vi "Autonomous Independent.vi"() -> ()   [LabVIEW 2020]
doc: "This VI is called when autonomous begins, and will automatically be terminated when autonomous ends. You can carry out timed or sensor driven robot movement independently without needing to return to the caller."
uses:
  <vilib>/Rock Robotics/WPI/Utilities/WPI_GetSetVariantRefNum.vi
  <vilib>/Rock Robotics/Network Tables/NT Write Numeric Array.vi
  Robot Global Data.vi
  <vilib>/Rock Robotics/Network Tables/NT Read String.vi
  <vilib>/Rock Robotics/WPI/RobotDrive/WPI_RobotDriveArcadeDrive_Standard(NoSaturation).vi
  <vilib>/Rock Robotics/WPI/ThirdParty/JAS_Junk/TrajLib/Trajectory_Library.lvlib
panel:
  out "Current Movement, for debugging":T1 {"Y Joystick Value" scale=1.0..-1.0; "X Joystick Value" scale=-1.0..1.0}
  in  "Array of robot movements":T2(array[cluster])=[{"X Joystick Value"=0.39393939393939403, "Y Joystick Value"=0.0, "Delay (sec)"=1.0, "Movement Name"="turn"}, {"X Joystick Value"=-0.3737373737373737, "Y Joystick Value"=0.0, "Delay (sec)"=1.0, "Movement Name"="turn back"}] {"Y Joystick Value" scale=1.0..-1.0; "X Joystick Value" scale=-1.0..1.0}
  # "Be sure to right-click and choose Data Operations>>Make Current Value default if you want to save the array values with the VI"
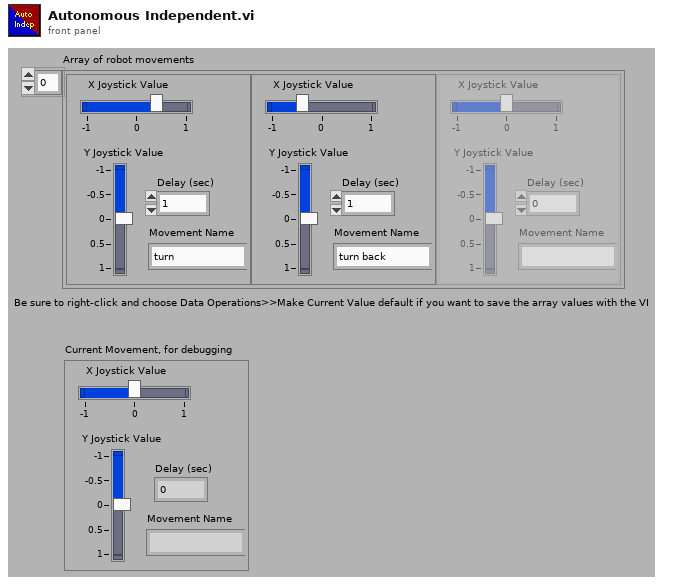
[diagram p1: front panel]
types:
  T1 = cluster{"X Joystick Value":dbl, "Y Joystick Value":dbl, "Delay (sec)":dbl, "Movement Name":string}
  T2 = cluster{"X Joystick Value":dbl, "Y Joystick Value":dbl, "Delay (sec)":dbl, "Movement Name":string}[]
  T3 = typedef "WPI_JoystickDevRef.ctl" = cluster{"Device":T4}
  T4 = typedef "WPI_JoystickDeviceEnum.ctl" = enum16{"USB 0", "USB 1", "USB 2", "USB 3", "USB 4", "USB 5"}
  T5 = typedef "Trajectory_Library.lvlib/SWERVE_DRIVE_ODOMETRY.ctl" = cluster{"POSE":T6, "GyroOffset":T8, "PreviousAngle":T8, "PrevModulePositions":T9[], "NumModules":i32}
  T6 = typedef "Trajectory_Library.lvlib/POSE2D.ctl" = cluster{"TRANSLATION":T7, "ROTATION":T8}
  T7 = typedef "Trajectory_Library.lvlib/TRANSLATION2D.ctl" = cluster{"X":dbl, "Y":dbl}
  T8 = typedef "Trajectory_Library.lvlib/ROTATION2D.ctl" = cluster{"VALUE":dbl, "COS":dbl, "SIN":dbl}
  T9 = typedef "Trajectory_Library.lvlib/SWERVE_DRIVE_MODULE_POSITION.ctl" = cluster{"Distance":dbl, "Angle":T8, "P":bool}
  T10 = typedef "WPI_RobotDriveDevRef.ctl" = cluster{"DevStatus":errorcluster, "Motors[]":T11[], "Square Inputs":bool, "Max Output":dbl}
  T11 = typedef "WPI_MotorControlDeviceRef.ctl" = cluster{"DeviceStatus":errorcluster, "Type":T12, "PWM":cluster{"PWM Channel":T13, "DeadBand":T14}, "CAN":cluster{"Device Number":u8, "SetOutput VI Ref":variant, "GetOutput VI Ref":variant, "Enable VI Ref":variant, "Disable VI Ref":variant, "Data":variant}, "Invert":bool, "DIO PWM":cluster{"PWM \"Enable\" Channel":T13, "DIOChannel":T15, "PWM Rate":dbl}}
  T12 = typedef "WPI_MotorControlType.ctl" = enum16{"PWM", "CAN", "DIO PWM"}
  T13 = typedef "FPGA_DIOPWMChannel.ctl" = enum8{"PWM 0", "PWM 1", "PWM 2", "PWM 3", "PWM 4", "PWM 5", "PWM 6", "PWM 7", "PWM 8", "PWM 9", "PWM MXP 0", "PWM MXP 1", "PWM MXP 2", "PWM MXP 3", "PWM MXP 4", "PWM MXP 5", "PWM MXP 6", "PWM MXP 7", "PWM MXP 8", "PWM MXP 9", "Invalid"}
  T14 = typedef "WPI_PWMDeadband.ctl" = cluster{"Name":string, "maxPositivePwm":i32, "minPositivePwm":i32, "centerPwm":i32, "maxNegativePwm":i32, "minNegativePwm":i32, "angularRange":u16}
  T15 = typedef "FPGA_DIOChannel.ctl" = enum8{"DIO 0", "DIO 1", "DIO 2", "DIO 3", "DIO 4", "DIO 5", "DIO 6", "DIO 7", "DIO 8", "DIO 9", "DIO MXP 0", "DIO MXP 1", "DIO MXP 2", "DIO MXP 3", "DIO MXP 4", "DIO MXP 5", "DIO MXP 6", "DIO MXP 7", "DIO MXP 8", "DIO MXP 9", "DIO MXP 10", "DIO MXP 11", "DIO MXP 12", "DIO MXP 13", "DIO MXP 14", "DIO MXP 15", "SPI Port CS1", "SPI Port CS2", "SPI Port CS3", "SPI Port MISO", "SPI Port MOSI", "Invalid"}
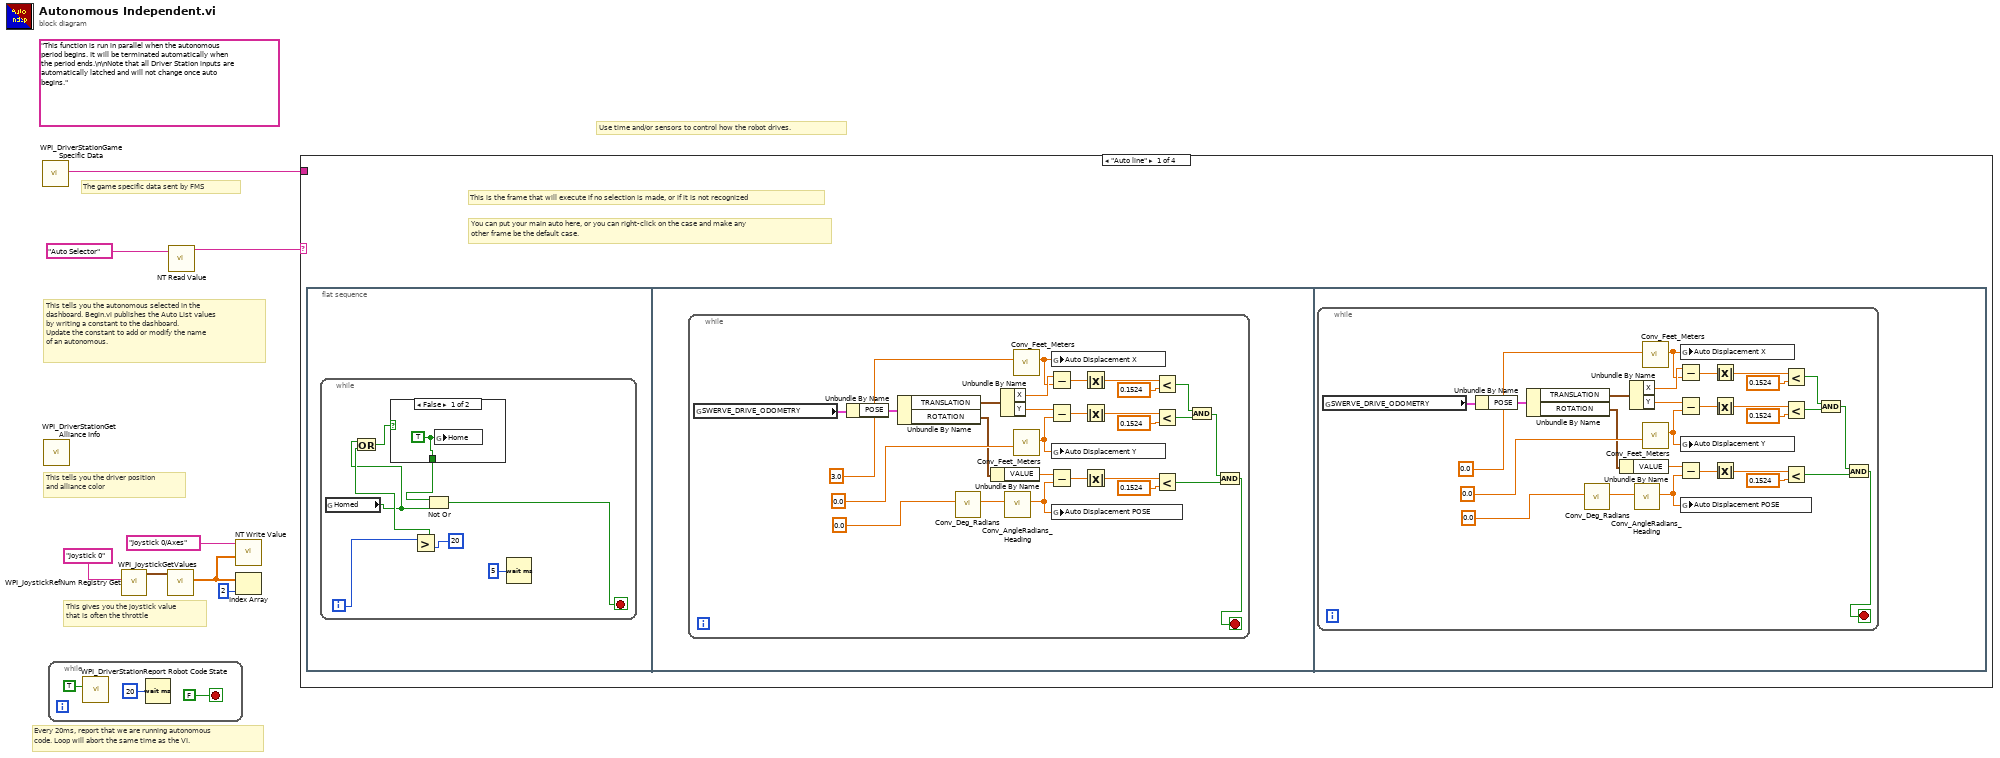
[diagram p0: block diagram]
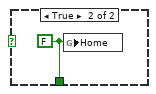
[diagram p2: hidden frame]
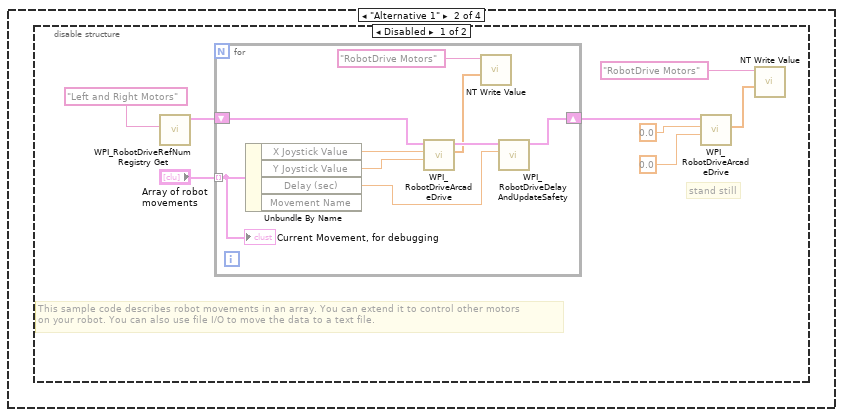
[diagram p3: hidden frame]
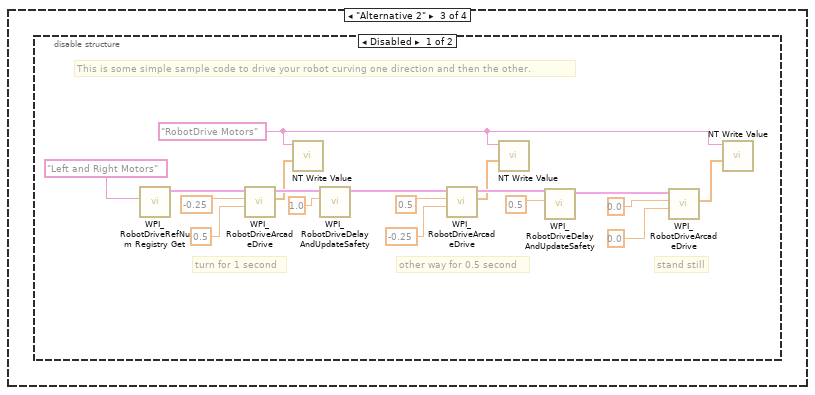
[diagram p5: hidden frame]
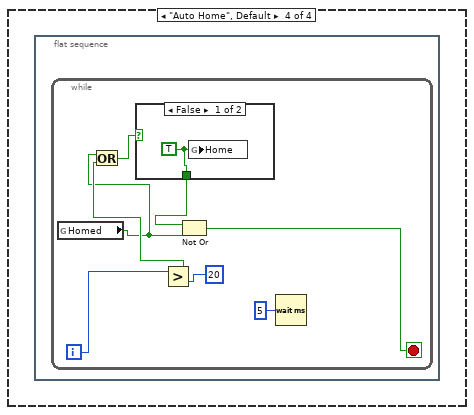
[diagram p7: hidden frame]
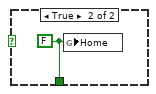
[diagram p8: hidden frame]
diagram:
  (unwired) "This function is run in parallel when the autonomous period begins. It will be terminated automatically when the period ends.\n\nNote that all Driver Station inputs are automatically latched and will not change once auto begins."
  # "The game specific data sent by FMS"
  # "This tells you the autonomous selected in the \ndashboard. Begin.vi publishes the Auto List values\nby writing a constant to the dashboard.\nUpdate the constant to add or modify the name\nof an autonomous."
  # "Every 20ms, report that we are running autonomous\ncode. Loop will abort the same time as the VI."
  # "This gives you the joystick value\nthat is often the throttle"
  # "Use time and/or sensors to control how the robot drives."
  # "This tells you the driver position\nand alliance color"
  n1 = call <vilib>:"WPI_DriverStationGame Specific Data.vi"() -> ("Game Specific Data"=w1:string)  [unwired: 11 in]
  n2 = call <vilib>:"WPI_DriverStationGet Alliance Info.vi"() -> ()  [unwired: 12 out]
  n3 = while {
    stop <- FALSE stop-if-true
    n4 = call <vilib>:"WPI_DriverStationReport Robot Code State.vi"("Autonomous"=TRUE) -> ()  [unwired: 10 in, 1 out]
    n5 = Wait (ms)(milliseconds to wait=u32 20) -> ()  [unwired: 1 out]
  }
  n6 = call <vilib>:"WPI_JoystickRefNum Registry Get.vi"("refnum name"="Joystick 0") -> ("JoystickDevRef"=w7:T3)  [unwired: 1 in, 9 out]
  n7 = call <vilib>:"WPI_JoystickGetValues.vi"("JoystickDevRef"=w7) -> ("Axes"=w3:dbl[])  [unwired: 6 in, 4 out]
  n8 = call-poly <vilib>:"NT Read Value.vi"("name"="Auto Selector" ("Name")) -> ("value"=w4:string)  [unwired: 8 in, 2 out]
  n9 = call-poly <vilib>:"NT Write Value.vi"("value"=w3, "name"="Joystick 0/Axes" ("Name")) -> ()  [unwired: 9 in, 1 out]
  n10 = Index Array(array=w3, index=2) -> ()  [unwired: 1 out]
  n11 = case shown="\"Auto line\"" w4 {
    tunnel: w1 -> [_ _ _ _]
    frame "Auto line" {
      # "You can put your main auto here, or you can right-click on the case and make any\nother frame be the default case."
      # "This is the frame that will execute if no selection is made, or if it is not recognized"
      n12 = flat-sequence {
        frame #0 {
          n13 = while {
            i -> [w17]
            stop <- w18 stop-if-true
            n14 = global read "Robot Global Data.vi" "Homed"() -> (w12:bool)
            n15 = Greater?(x=w17, y=20) -> (0:w13:bool)
            n16 = Or(x=w12, y=w13) -> (x .or. y?=w14:bool)
            n17 = case shown="False" w14 {
              tunnel: [w20 w21] -> w19
              frame False {
                w20 = TRUE ("Homed")
                n18 = global write "Robot Global Data.vi" "Home"(w20) -> ()
              }
              frame True {
                w21 = FALSE ("Homed")
                n19 = global write "Robot Global Data.vi" "Home"(w21) -> ()
              }
            }
            n20 = Not Or(1:w12, 2:w19) -> (0:w18:bool)
            n21 = Wait (ms)(milliseconds to wait=u32 5) -> ()  [unwired: 1 out]
          }
        }
        frame #1 {
          n22 = while {
            stop <- w28 stop-if-true
            n23 = global read "Robot Global Data.vi" "SWERVE_DRIVE_ODOMETRY"() -> (w45:T5)
            n24 = Unbundle By Name(w45) -> ("POSE"=w44:T6)
            n25 = Unbundle By Name(w44) -> ("TRANSLATION"=w43:T7, "ROTATION"=w42:T8)
            n26 = call <vilib>:"Conv_Deg_Radians.vi"("Degress"=0.0) -> ("Radians"=w46:dbl)  [unwired: 10 in]
            n27 = Unbundle By Name(w42) -> ("VALUE"=w31:dbl)
            n28 = Unbundle By Name(w43) -> ("X"=w40:dbl, "Y"=w33:dbl)
            n29 = call <vilib>:"Conv_AngleRadians_Heading.vi"("Radians"=w46) -> ("Heading"=w30:dbl)  [unwired: 10 in]
            n30 = call <vilib>:"Conv_Feet_Meters.vi"("Feet"=3.0) -> ("Meters"=w39:dbl)  [unwired: 10 in]
            n31 = call <vilib>:"Conv_Feet_Meters.vi"("Feet"=0.0) -> ("Meters"=w32:dbl)  [unwired: 10 in]
            n32 = Subtract(x=w40, y=w39) -> (x-y=w41:dbl)
            n33 = Subtract(x=w33, y=w32) -> (x-y=w36:dbl)
            n34 = Subtract(x=w31, y=w30) -> (x-y=w35:dbl)
            n35 = global write "Robot Global Data.vi" "Auto Displacement X"(w39) -> ()
            n36 = global write "Robot Global Data.vi" "Auto Displacement Y"(w32) -> ()
            n37 = global write "Robot Global Data.vi" "Auto Displacement POSE"(w30) -> ()
            n38 = Absolute Value(x=w41) -> (abs(x)=w24:dbl)
            n39 = Absolute Value(x=w36) -> (abs(x)=w23:dbl)
            n40 = Absolute Value(x=w35) -> (abs(x)=w22:dbl)
            n41 = Less?(x=w24, y=0.1524) -> (x < y?=w27:bool)
            n42 = Less?(x=w23, y=0.1524) -> (x < y?=w26:bool)
            n43 = Less?(x=w22, y=0.1524) -> (x < y?=w25:bool)
            n44 = And(x=w27, y=w26) -> (x .and. y?=w29:bool)
            n45 = And(x=w29, y=w25) -> (x .and. y?=w28:bool)
          }
        }
        frame #2 {
          n46 = while {
            stop <- w56 stop-if-true
            n47 = global read "Robot Global Data.vi" "SWERVE_DRIVE_ODOMETRY"() -> (w73:T5)
            n48 = Unbundle By Name(w73) -> ("POSE"=w72:T6)
            n49 = Unbundle By Name(w72) -> ("TRANSLATION"=w71:T7, "ROTATION"=w70:T8)
            n50 = call <vilib>:"Conv_Deg_Radians.vi"("Degress"=0.0) -> ("Radians"=w74:dbl)  [unwired: 10 in]
            n51 = Unbundle By Name(w70) -> ("VALUE"=w59:dbl)
            n52 = Unbundle By Name(w71) -> ("X"=w68:dbl, "Y"=w61:dbl)
            n53 = call <vilib>:"Conv_AngleRadians_Heading.vi"("Radians"=w74) -> ("Heading"=w58:dbl)  [unwired: 10 in]
            n54 = call <vilib>:"Conv_Feet_Meters.vi"("Feet"=0.0) -> ("Meters"=w67:dbl)  [unwired: 10 in]
            n55 = call <vilib>:"Conv_Feet_Meters.vi"("Feet"=0.0) -> ("Meters"=w60:dbl)  [unwired: 10 in]
            n56 = Subtract(x=w68, y=w67) -> (x-y=w69:dbl)
            n57 = Subtract(x=w61, y=w60) -> (x-y=w64:dbl)
            n58 = Subtract(x=w59, y=w58) -> (x-y=w63:dbl)
            n59 = global write "Robot Global Data.vi" "Auto Displacement X"(w67) -> ()
            n60 = global write "Robot Global Data.vi" "Auto Displacement Y"(w60) -> ()
            n61 = global write "Robot Global Data.vi" "Auto Displacement POSE"(w58) -> ()
            n62 = Absolute Value(x=w69) -> (abs(x)=w52:dbl)
            n63 = Absolute Value(x=w64) -> (abs(x)=w51:dbl)
            n64 = Absolute Value(x=w63) -> (abs(x)=w50:dbl)
            n65 = Less?(x=w52, y=0.1524) -> (x < y?=w55:bool)
            n66 = Less?(x=w51, y=0.1524) -> (x < y?=w54:bool)
            n67 = Less?(x=w50, y=0.1524) -> (x < y?=w53:bool)
            n68 = And(x=w55, y=w54) -> (x .and. y?=w57:bool)
            n69 = And(x=w57, y=w53) -> (x .and. y?=w56:bool)
          }
        }
      }
    }
    frame "Alternative 1" {
      n70 = disable-structure shown="Disabled" {
        frame Disabled {
          # "stand still"
          # "This sample code describes robot movements in an array. You can extend it to control other motors\non your robot. You can also use file I/O to move the data to a text file."
          n71 = call <vilib>:"WPI_RobotDriveRefNum Registry Get.vi"("refnum name"="Left and Right Motors") -> ("RobotDriveDevRef"=w84:T10)  [unwired: 1 in, 9 out]
          n72 = for {
            shift-right: [w92] -> w79
            shift-left: w84 -> [w93]
            tunnel: "Array of robot movements" -> [w88] mode=indexing
            n73 = Unbundle By Name(w88) -> ("X Joystick Value"=w91:dbl, "Y Joystick Value"=w90:dbl, "Delay (sec)"=w89:dbl)  [unwired: 1 out]
            n74 = call-poly <vilib>:"WPI_RobotDriveArcadeDrive.vi"("Y axis value"=w90, "X axis value"=w91, "RobotDriveDevRef"=w93) -> ("Motor Values"=w86:dbl[], "RobotDriveDevRef"=w94:T10)  [unwired: 1 in, 6 out]
            n75 = call-poly <vilib>:"NT Write Value.vi"("value"=w86, "name"="RobotDrive Motors" ("Name")) -> ()  [unwired: 9 in, 1 out]
            n76 = call <vilib>:"WPI_RobotDriveDelayAndUpdateSafety.vi"("Delay (s)"=w89, "RobotDriveDevRef"=w94) -> ("RobotDriveDevRef 2"=w92:T10)  [unwired: 8 in, 1 out]
            "Current Movement, for debugging" <- w88
          }
          n77 = call-poly <vilib>:"WPI_RobotDriveArcadeDrive.vi"("Y axis value"=0.0 ("X axis value"), "X axis value"=0.0, "RobotDriveDevRef"=w79) -> ("Motor Values"=w82:dbl[])  [unwired: 1 in, 7 out]
          n78 = call-poly <vilib>:"NT Write Value.vi"("value"=w82, "name"="RobotDrive Motors" ("Name")) -> ()  [unwired: 9 in, 1 out]
        }
        frame Enabled {
        }
      }
    }
    frame "Alternative 2" {
      n79 = disable-structure shown="Disabled" {
        frame Disabled {
          w96 = "RobotDrive Motors" ("Name")
          # "This is some simple sample code to drive your robot curving one direction and then the other."
          # "stand still"
          # "other way for 0.5 second"
          # "turn for 1 second"
          n80 = call <vilib>:"WPI_RobotDriveRefNum Registry Get.vi"("refnum name"="Left and Right Motors") -> ("RobotDriveDevRef"=w112:T10)  [unwired: 1 in, 9 out]
          n81 = call-poly <vilib>:"WPI_RobotDriveArcadeDrive.vi"("Y axis value"=0.5 ("X axis value"), "X axis value"=-0.25, "RobotDriveDevRef"=w112) -> ("Motor Values"=w95:dbl[], "RobotDriveDevRef"=w105:T10)  [unwired: 1 in, 6 out]
          n82 = call-poly <vilib>:"NT Write Value.vi"("value"=w95, "name"=w96) -> ()  [unwired: 9 in, 1 out]
          n83 = call <vilib>:"WPI_RobotDriveDelayAndUpdateSafety.vi"("Delay (s)"=1.0, "RobotDriveDevRef"=w105) -> ("RobotDriveDevRef 2"=w106:T10)  [unwired: 8 in, 1 out]
          n84 = call-poly <vilib>:"WPI_RobotDriveArcadeDrive.vi"("Y axis value"=-0.25 ("X axis value"), "X axis value"=0.5, "RobotDriveDevRef"=w106) -> ("Motor Values"=w97:dbl[], "RobotDriveDevRef"=w107:T10)  [unwired: 1 in, 6 out]
          n85 = call-poly <vilib>:"NT Write Value.vi"("value"=w97, "name"=w96) -> ()  [unwired: 9 in, 1 out]
          n86 = call <vilib>:"WPI_RobotDriveDelayAndUpdateSafety.vi"("Delay (s)"=0.5, "RobotDriveDevRef"=w107) -> ("RobotDriveDevRef 2"=w108:T10)  [unwired: 8 in, 1 out]
          n87 = call-poly <vilib>:"WPI_RobotDriveArcadeDrive.vi"("Y axis value"=0.0 ("X axis value"), "X axis value"=0.0, "RobotDriveDevRef"=w108) -> ("Motor Values"=w98:dbl[])  [unwired: 1 in, 7 out]
          n88 = call-poly <vilib>:"NT Write Value.vi"("value"=w98, "name"=w96) -> ()  [unwired: 9 in, 1 out]
        }
        frame Enabled {
        }
      }
    }
    frame "Auto Home", Default {
      n89 = flat-sequence {
        frame #0 {
          n90 = while {
            i -> [w118]
            stop <- w119 stop-if-true
            n91 = global read "Robot Global Data.vi" "Homed"() -> (w113:bool)
            n92 = Greater?(x=w118, y=20) -> (0:w114:bool)
            n93 = Or(x=w113, y=w114) -> (x .or. y?=w115:bool)
            n94 = case shown="False" w115 {
              tunnel: [w121 w122] -> w120
              frame False {
                w121 = TRUE ("Homed")
                n95 = global write "Robot Global Data.vi" "Home"(w121) -> ()
              }
              frame True {
                w122 = FALSE ("Homed")
                n96 = global write "Robot Global Data.vi" "Home"(w122) -> ()
              }
            }
            n97 = Not Or(1:w113, 2:w120) -> (0:w119:bool)
            n98 = Wait (ms)(milliseconds to wait=u32 5) -> ()  [unwired: 1 out]
          }
        }
      }
    }
  }
